vi "HEWH Message Filter.vi"(7 "Main Display?":bool, 8 "Error In":errorcluster, 10 "Station Message":string, 11 "Main Message":string) -> (0 "Error Out":errorcluster, 3 "Combined Message":string)   [LabVIEW 2016]
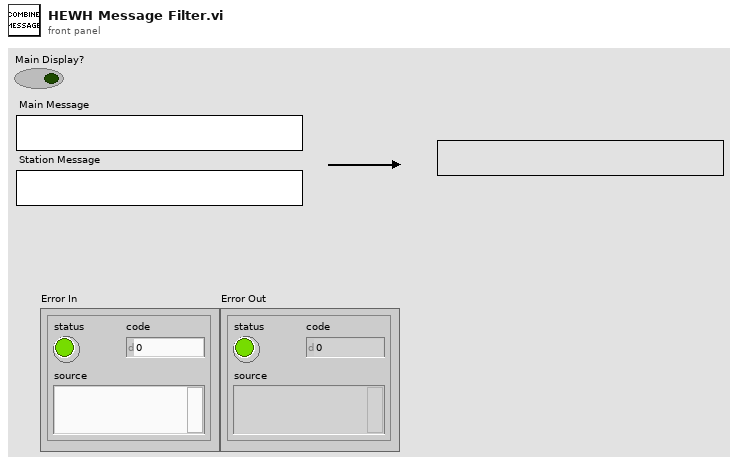
[diagram p1: front panel]
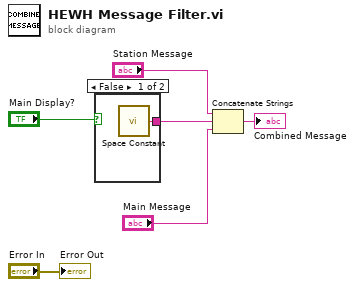
[diagram p0: block diagram]
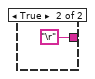
[diagram p2: hidden frame]
diagram:
  n1 = case shown="False" "Main Display?" {
    tunnel: [w7 "\r"] -> w1
    frame False {
      n2 = call <vilib>:"Space Constant.vi"() -> ("String"=w7:string)
    }
    frame True {
    }
  }
  n3 = Concatenate Strings("Station Message", w1, "Main Message") -> (→"Combined Message":string)
  "Error Out" <- "Error In"
